vi "Update Descriptions.vi"() -> ()   [LabVIEW 2013]
uses:
  <vilib>/xml/Load XML File.vi
  <vilib>/xml/Close Reference(Node).vi
  <vilib>/xml/Close Reference(NNMap).vi
  <vilib>/xml/NI_XML.lvlib
  <resource>/objmgr/DOMUserDefRef.rc
panel:
  out "error out":errorcluster
  in  "Path":path=path "../lvssh2-descriptions.xml"
  # "When executed, takes the titles and descriptions from file and applies them\nto the corresponding VI."
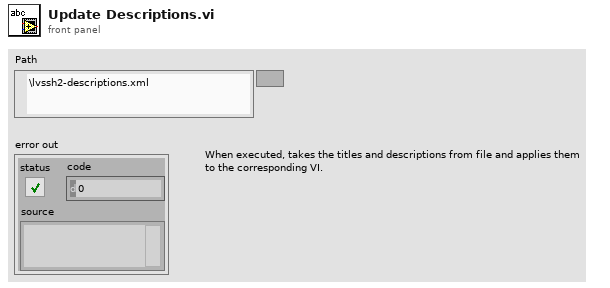
[diagram p1: front panel]
types:
  T1 = cluster{"path":string, "title":string, "description":string}
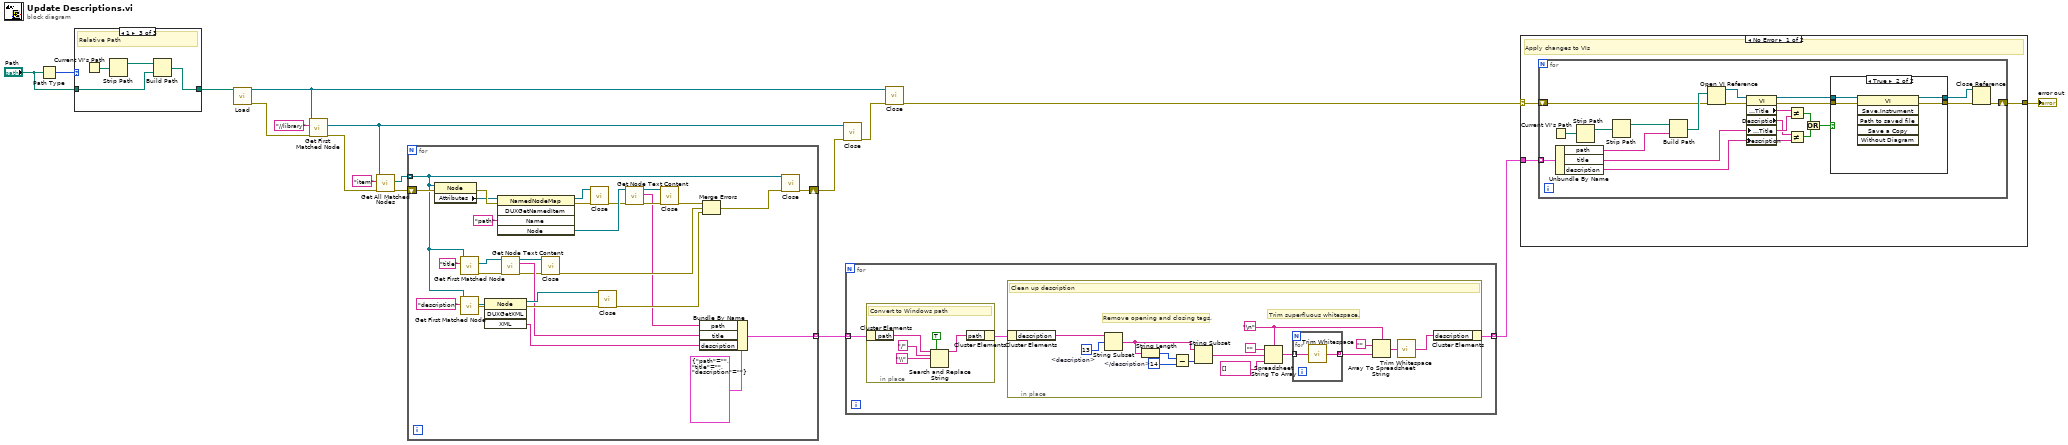
[diagram p0: block diagram]
diagram:
  n1 = Path Type(1:"Path") -> (0:w17:i16)
  n2 = case shown="1" w17 {
    tunnel: "Path" -> [_ w18 w19]
    tunnel: [_ w18 w22] -> w15
    frame Default {
      # "<Not A Path>"
    }
    frame 0 {
      # "Absolute Path"
    }
    frame 1 {
      # "Relative Path"
      n3 = Current VI's Path() -> (path=w21:path)
      n4 = Strip Path(path=w21) -> (stripped path=w20:path)  [unwired: 1 out]
      n5 = Build Path(base path=w20, name or relative path=w19) -> (appended path=w22:path)
    }
  }
  n6 = call-poly <vilib>:"Load.vi"("path to XML document"=w15) -> ("DOM document out"=w14:refnum<k20>, "error out"=w12:errorcluster)  [unwired: 12 in, 1 out]
  n7 = call <vilib>:"Get First Matched Node.vi"("error in (no error)"=w12, "XPath expression"="//library", "node in"=w14) -> ("error out"=w10:errorcluster, "node result"=w6:refnum<k20>)  [unwired: 6 in, 1 out]
  n8 = call <vilib>:"Get All Matched Nodes.vi"("error in (no error)"=w10, "XPath expression"="item", "node in"=w6) -> ("error out"=w8:errorcluster, "node result array"=w5:refnum<k20>[])  [unwired: 6 in, 1 out]
  n9 = for {
    tunnel: w5 -> [w40] mode=indexing
    shift-right: [w53] -> w9
    shift-left: w8 -> [w52]
    tunnel: [w45] -> w1 mode=indexing
    n10 = property class="Node"(reference=w40, error in=w52) -> (error out=w51:errorcluster, "Attributes"=w48:refnum<k20>)  [unwired: 1 out]
    n11 = call <vilib>:"Get First Matched Node.vi"("XPath expression"="title", "node in"=w40) -> ("error out"=w28:errorcluster, "node result"=w38:refnum<k20>)  [unwired: 7 in, 1 out]
    n12 = call <vilib>:"Get First Matched Node.vi"("XPath expression"="description", "node in"=w40) -> ("error out"=w37:errorcluster, "node result"=w36:refnum<k20>)  [unwired: 7 in, 1 out]
    n13 = invoke class="Node" method="DUXGetXML"(reference=w36, error in=w37) -> (reference out=w35:refnum<k20>, error out=w34:errorcluster, "XML"=w25:string)  [unwired: 2 in, 1 out]
    n14 = invoke class="NamedNodeMap" method="DUXGetNamedItem"(reference=w48, error in=w51, "Name"="path") -> (reference out=w47:refnum<k20>, error out=w49:errorcluster, "Node"=w44:refnum<k20>)  [unwired: 2 in, 2 out]
    n15 = call <vilib>:"Get Node Text Content.vi"("error in (no error)"=w28, "node in"=w38) -> ("error out"=w26:errorcluster, "node text"=w27:string, "node out"=w33:refnum<k20>)  [unwired: 7 in]
    n16 = call-poly <vilib>:"Close.vi"("error in (no error)"=w26, "node"=w33) -> ("error out"=w32:errorcluster)  [unwired: 7 in]
    n17 = call-poly <vilib>:"Close.vi"("error in (no error)"=w49, "named node map"=w47) -> ("error out"=w43:errorcluster)  [unwired: 7 in]
    n18 = call-poly <vilib>:"Close.vi"("error in (no error)"=w34, "node"=w35) -> ("error out"=w31:errorcluster)  [unwired: 7 in]
    n19 = call <vilib>:"Get Node Text Content.vi"("error in (no error)"=w43, "node in"=w44) -> ("error out"=w42:errorcluster, "node text"=w24:string, "node out"=w41:refnum<k20>)  [unwired: 7 in]
    n20 = call-poly <vilib>:"Close.vi"("error in (no error)"=w42, "node"=w41) -> ("error out"=w30:errorcluster)  [unwired: 7 in]
    n21 = Bundle By Name(cluster=T1 {"path"="", "title"="", "description"=""}, "path"=w24, "title"=w27, "description"=w25) -> (w45:T1)
    n22 = Merge Errors(w30, w32, w31) -> (w29:errorcluster)
    n23 = call-poly <vilib>:"Close.vi"("error in (no error)"=w29, "node"=w40) -> ("error out"=w53:errorcluster)  [unwired: 7 in]
  }
  n24 = call-poly <vilib>:"Close.vi"("error in (no error)"=w9, "node"=w6) -> ("error out"=w11:errorcluster)  [unwired: 7 in]
  n25 = for {
    tunnel: [w54] -> w2 mode=indexing
    tunnel: w1 -> [w56] mode=indexing
    n26 = in-place {
      # "Convert to Windows path"
      n27 = in-place-cluster #1(w56) -> ("path"=w75:string)
      n28 = Search and Replace String(replace all?=TRUE ("replace all? (F)"), input string=w75, search string="/", replace string="\\" ("replace string (\"\")")) -> (result string=w74:string)  [unwired: 4 in, 3 out]
      n29 = in-place-cluster #1("path"=w74) -> (w55:T1)
    }
    n30 = in-place {
      w64 = "\n"
      w61 = 14  # </description>
      w60 = 13  # <description>
      # "Trim superfluous whitespace."
      # "Remove opening and closing tags."
      # "Clean up description"
      n31 = in-place-cluster #2(w55) -> ("description"=w62:string)
      n32 = String Subset(string=w62, offset (0)=w60) -> (substring=w71:string)  [unwired: 1 in]
      n33 = String Length(string=w71) -> (length=w70:i32)
      n34 = Subtract(x=w70, y=w61) -> (x-y=w69:i32)
      n35 = String Subset(string=w71, length (rest)=w69) -> (substring=w68:string)  [unwired: 1 in]
      n36 = Spreadsheet String To Array(delimiter (Tab)=w64, format string="", spreadsheet string=w68, array type (2D Dbl)=string[] []) -> (array=w66:string[])
      n37 = for {
        tunnel: w66 -> [w73] mode=indexing
        tunnel: [w72] -> w65 mode=indexing
        n38 = call <vilib>:"Trim Whitespace.vi"("string"=w73) -> ("trimmed string"=w72:string)  [unwired: 1 in]
      }
      n39 = Array To Spreadsheet String(delimiter (Tab)=w64, array=w65, 3:"") -> (spreadsheet string=w58:string)
      n40 = call <vilib>:"Trim Whitespace.vi"("string"=w58) -> ("trimmed string"=w57:string)  [unwired: 1 in]
      n41 = in-place-cluster #2("description"=w57) -> (w54:T1)
    }
  }
  n42 = call-poly <vilib>:"Close.vi"("error in (no error)"=w11, "node"=w14) -> ("error out"=w4:errorcluster)  [unwired: 7 in]
  n43 = case shown="No Error" w4 {
    selector: w4 -> [w79 w109]
    tunnel: [w80 w109] -> w3
    tunnel: w2 -> [w81 _]
    frame No Error {
      # "Apply changes to VIs"
      n44 = for {
        tunnel: w81 -> [w102] mode=indexing
        shift-right: [w94] -> w80
        shift-left: w79 -> [w93]
        n45 = Current VI's Path() -> (path=w92:path)
        n46 = Unbundle By Name(w102) -> ("path"=w91:string, "title"=w90:string, "description"=w88:string)
        n47 = Strip Path(path=w92) -> (stripped path=w83:path)  [unwired: 1 out]
        n48 = Strip Path(path=w83) -> (stripped path=w82:path)  [unwired: 1 out]
        n49 = Build Path(base path=w82, name or relative path=w91) -> (appended path=w101:path)
        n50 = Open VI Reference(vi path=w101, error in (no error)=w93) -> (vi reference=w100:refnum<vi>, error out=w99:errorcluster)  [unwired: 4 in]
        n51 = property class="VI"(reference=w100, error in=w99, "Front Panel.Title"=w90, "Description"=w88) -> (reference out=w97:refnum<vi>, error out=w98:errorcluster, "Front Panel.Title"=w89:string, "Description"=w87:string)
        n52 = Not Equal?(x=w89, y=w90) -> (x != y?=w86:bool)
        n53 = Not Equal?(x=w87, y=w88) -> (x != y?=w85:bool)
        n54 = Or(x=w86, y=w85) -> (x .or. y?=w84:bool)
        n55 = case shown="True" w84 {
          tunnel: w98 -> [w104 w108]
          tunnel: w97 -> [w103 w107]
          tunnel: [w104 w106] -> w96
          tunnel: [w103 w105] -> w95
          frame False {
          }
          frame True {
            n56 = invoke class="VI" method="Save.Instrument"(reference=w107, error in=w108) -> (reference out=w105:refnum<vi>, error out=w106:errorcluster)  [unwired: 4 in, 4 out]
          }
        }
        n57 = Close Reference(reference=w95, error in (no error)=w96) -> (error out=w94:errorcluster)
      }
    }
    frame Error {
    }
  }
  "error out" <- w3
